vi "parse_gripper_state.vi"(4 "error in":errorcluster, 7 "msg in":string="\u0001\u0001\u0001\u0000\u0000\u0000\u0000\b‚uÀBff\u0006A") -> (0 "error out":errorcluster, 2 "Gripper State":T1, 3 "msg out":string)   [LabVIEW 2012]
uses:
  <userlib>/rosforlv/ROS/parsing/std_msgs/subs/parse_u8_scalar.vi
  <userlib>/rosforlv/ROS/parsing/std_msgs/subs/parse_float32_scalar.vi
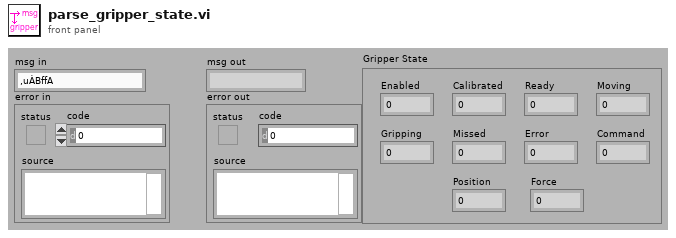
[diagram p1: front panel]
types:
  T1 = cluster{"Enabled":u8, "Calibrated":u8, "Ready":u8, "Moving":u8, "Gripping":u8, "Missed":u8, "Error":u8, "Command":u8, "Position":sgl, "Force":sgl}
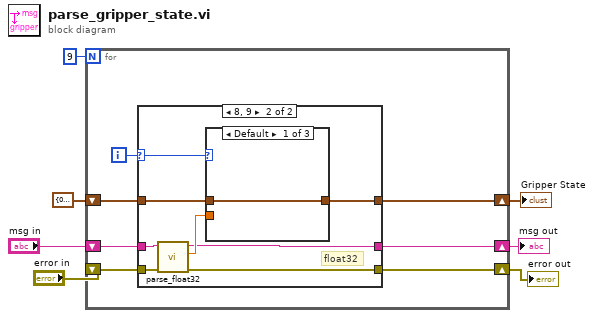
[diagram p0: block diagram]
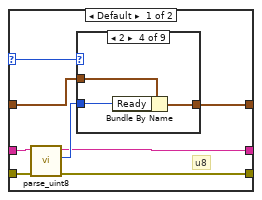
[diagram p2: hidden frame]
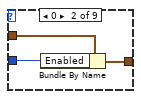
[diagram p4: hidden frame]
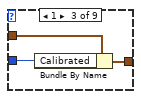
[diagram p5: hidden frame]
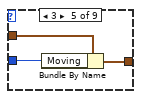
[diagram p6: hidden frame]
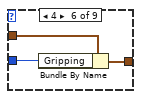
[diagram p7: hidden frame]
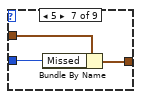
[diagram p8: hidden frame]
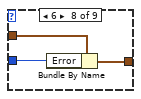
[diagram p9: hidden frame]
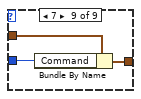
[diagram p10: hidden frame]
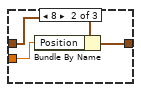
[diagram p11: hidden frame]
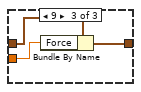
[diagram p12: hidden frame]
diagram:
  n1 = for {
    N: 9 -> [_]
    shift-right: [w10] -> w4
    shift-left: "msg in" -> [w13]
    shift-right: [w11] -> w6
    shift-left: T1 {"Enabled"=0, "Calibrated"=0, "Ready"=0, "Moving"=0, "Gripping"=0, "Missed"=0, "Error"=0, "Command"=0, "Position"=0.0, "Force"=0.0} ("Cluster") -> [w12]
    shift-right: [w8] -> w1
    shift-left: "error in" -> [w9]
    i -> [w14]
    n2 = case shown="8, 9" w14 {
      selector: w14 -> [w22 w55]
      tunnel: w13 -> [w17 w52]
      tunnel: [w18 w50] -> w10
      tunnel: w12 -> [w21 w54]
      tunnel: [w20 w53] -> w11
      tunnel: w9 -> [w16 w48]
      tunnel: [w15 w49] -> w8
      frame Default {
        # "u8"
        n3 = call-poly <userlib>:"parse_uint8.vi"("error in"=w16, "msg in"=w17) -> ("error out"=w15:errorcluster, "number"=w19:u8, "msg out"=w18:string)  [unwired: 3 in]
        n4 = case shown="2" w22 {
          tunnel: w19 -> [_ w24 w28 w31 w34 w37 w40 w43 w46]
          tunnel: w21 -> [w23 w26 w29 w32 w35 w38 w41 w44 w47]
          tunnel: [w23 w25 w27 w30 w33 w36 w39 w42 w45] -> w20
          frame Default {
          }
          frame 0 {
            n5 = Bundle By Name(cluster=w26, "Enabled"=w24) -> (w25:T1)
          }
          frame 1 {
            n6 = Bundle By Name(cluster=w29, "Calibrated"=w28) -> (w27:T1)
          }
          frame 2 {
            n7 = Bundle By Name(cluster=w32, "Ready"=w31) -> (w30:T1)
          }
          frame 3 {
            n8 = Bundle By Name(cluster=w35, "Moving"=w34) -> (w33:T1)
          }
          frame 4 {
            n9 = Bundle By Name(cluster=w38, "Gripping"=w37) -> (w36:T1)
          }
          frame 5 {
            n10 = Bundle By Name(cluster=w41, "Missed"=w40) -> (w39:T1)
          }
          frame 6 {
            n11 = Bundle By Name(cluster=w44, "Error"=w43) -> (w42:T1)
          }
          frame 7 {
            n12 = Bundle By Name(cluster=w47, "Command"=w46) -> (w45:T1)
          }
        }
      }
      frame 8, 9 {
        # "float32"
        n13 = call-poly <userlib>:"parse_float32.vi"("error in"=w48, "msg in"=w52) -> ("error out"=w49:errorcluster, "number"=w51:sgl, "msg out"=w50:string)  [unwired: 3 in]
        n14 = case shown="Default" w55 {
          tunnel: w54 -> [w56 w59 w62]
          tunnel: [w56 w57 w60] -> w53
          tunnel: w51 -> [_ w58 w61]
          frame Default {
          }
          frame 8 {
            n15 = Bundle By Name(cluster=w59, "Position"=w58) -> (w57:T1)
          }
          frame 9 {
            n16 = Bundle By Name(cluster=w62, "Force"=w61) -> (w60:T1)
          }
        }
      }
    }
  }
  "Gripper State" <- w6
  "msg out" <- w4
  "error out" <- w1
